vi "Within Range.vi"(7 "Range +-":dbl=200.0 format="%#_13g", 9 "Current Value":dbl, 11 "Desired Value":dbl) -> (3 "Within range?":bool)   [LabVIEW 2014]
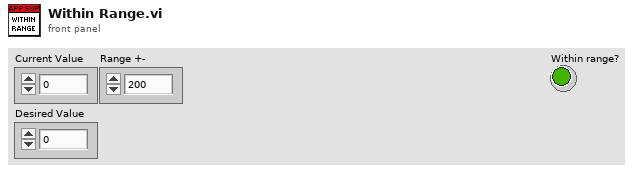
[diagram p1: front panel]
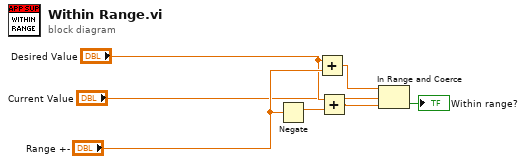
[diagram p0: block diagram]
diagram:
  n1 = Negate(x="Range +-") -> (-x=w7:dbl)
  n2 = Add(x="Desired Value", y="Range +-") -> (x+y=w4:dbl)
  n3 = Add(x="Desired Value", y=w7) -> (x+y=w5:dbl)
  n4 = In Range and Coerce(upper limit=w4, x="Current Value", lower limit=w5) -> (In Range?=→"Within range?":bool)  [unwired: 1 out]
